vi "TextIcon.vi"(0 "Text":u32(colorbox)=6589059, 1 "picture":picture, 5 "Text":string, 7 "[user-specified font]":T1={"Font Name:"="Arial", "Size"=6, "Strikeout?"=FALSE, "Italic?"=FALSE, "Underline?"=FALSE, "Outline?"=FALSE, "Shadow?"=FALSE, "Bold?"=FALSE}, 9 "rect":T3={"left"=2, "top"=17, "right"=32, "bottom"=32}, 11 "error in (no error)":errorcluster, 12 "BG color(transparent)":u32(colorbox)=16777216) -> (4 ">> TextIcon >>":T4 caption="用户图层", 15 "error out":errorcluster)   [LabVIEW 2015]
uses:
  <vilib>/LabVIEW Icon API/API_User Layer Data.ctl
  <vilib>/Utility/miscctls.llb/LVPoint32TypeDef.ctl
  <vilib>/picture/picture.llb/imagedata.ctl
  1_ctl/Ctl-Text-Set.ctl
  1_ctl/ctl-font.ctl
  <vilib>/LabVIEW Icon API/LabVIEW Icon API.lvlib
panel:
  out "picture 2":picture
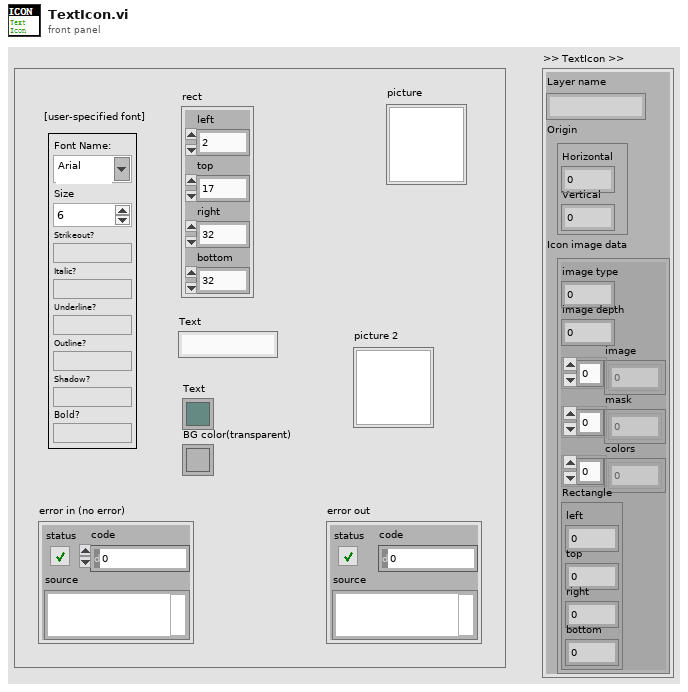
[diagram p1: front panel]
types:
  T1 = typedef "Ctl-Text-Set.ctl" = cluster{"Font Name:":T2, "Size":i16, "Strikeout?":bool, "Italic?":bool, "Underline?":bool, "Outline?":bool, "Shadow?":bool, "Bold?":bool}
  T2 = typedef "ctl-font.ctl" = string
  T3 = cluster{"left":i16, "top":i16, "right":i16, "bottom":i16}
  T4 = typedef "LabVIEW Icon API.lvlib/API_User Layer Data.ctl" = cluster{"Layer name":string, "Origin":T5, "Icon image data":T6}
  T5 = typedef "LVPoint32TypeDef.ctl" = cluster{"Horizontal":i32, "Vertical":i32}
  T6 = typedef "imagedata.ctl" = cluster{"image type":i32, "image depth":i32, "image":u8[], "mask":u8[], "colors":u32[], "Rectangle":cluster{"left":i16, "top":i16, "right":i16, "bottom":i16}}
  T7 = enum16{"User-specified Font", "Application Font", "System Font", "Dialog Font"}
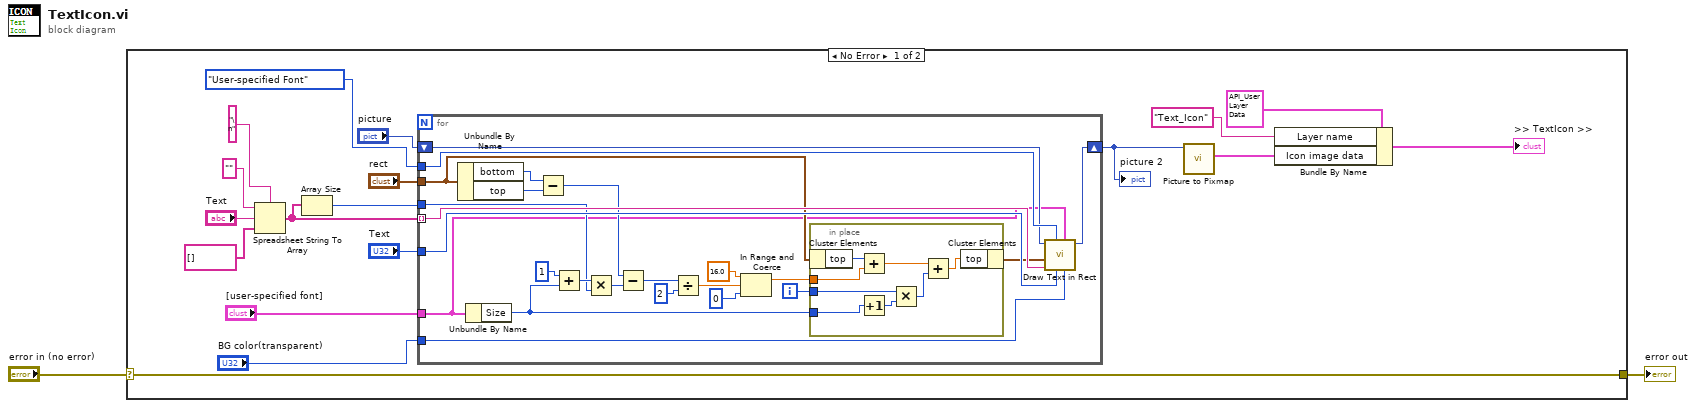
[diagram p0: block diagram]
diagram:
  n1 = case shown="No Error" "error in (no error)" {
    selector: "error in (no error)" -> [w7 w53]
    tunnel: [w7 w53] -> w1
    frame No Error {
      n2 = Spreadsheet String To Array(delimiter (Tab)="\n", format string="", spreadsheet string="Text", array type (2D Dbl)=string[] []) -> (array=w6:string[])
      n3 = Array Size(array=w6) -> (size(s)=w5:i32)
      n4 = for {
        tunnel: "Text" -> [w43]
        tunnel: "BG color(transparent)" -> [w42]
        tunnel: T7."User-specified Font" ("desired font(Application)") -> [w41]
        tunnel: "[user-specified font]" -> [w21]
        shift-right: [w44] -> w4
        shift-left: "picture" -> [w40]
        tunnel: w6 -> [w39] mode=indexing
        tunnel: "rect" -> [w36]
        tunnel: w5 -> [w29]
        i -> [w37]
        n5 = Unbundle By Name(w36) -> ("bottom"=w35:i16, "top"=w34:i16)
        n6 = Unbundle By Name(w21) -> ("Size"=w32:i16)
        n7 = Subtract(x=w35, y=w34) -> (x-y=w33:i16)
        n8 = Add(x=i16 1, y=w32) -> (x+y=w30:i16)
        n9 = Multiply(x=w30, y=w29) -> (x*y=w28:i32)
        n10 = Subtract(x=w33, y=w28) -> (x-y=w27:i32)
        n11 = Divide(x=w27, y=2) -> (x/y=w24:dbl)
        n12 = In Range and Coerce(upper limit=16.0, x=w24, lower limit=0 ("y")) -> (coerced(x)=w23:dbl)  [unwired: 1 out]
        n13 = in-place {
          in-place-border: w37 -> [w52]
          in-place-border: w32 -> [w50]
          in-place-border: w23 -> [w48]
          n14 = in-place-cluster #1(w36) -> ("top"=w46:i16)
          n15 = Add(x=w46, y=w48) -> (x+y=w47:dbl)
          n16 = Increment(x=w50) -> (x+1=w49:i16)
          n17 = Multiply(x=w52, y=w49) -> (x*y=w51:i32)
          n18 = Add(x=w47, y=w51) -> (x+y=w45:dbl)
          n19 = in-place-cluster #1("top"=w45) -> (w38:T3)
        }
        n20 = call <vilib>:"Draw Text in Rect.vi"("BG color(transparent)"=w42, "[user-specified font]"=w21, "text color(black)"=w43, "desired font(Application)"=w41, "text"=w39, "rect"=w38, "picture"=w40) -> ("new picture"=w44:picture)  [unwired: 4 in]
      }
      "picture 2" <- w4
      n21 = call <vilib>:"Picture to Pixmap.vi"("picture"=w4) -> ("image data"=w19:T6)  [unwired: 9 in, 1 out]
      n22 = Bundle By Name(cluster=T4 {"Layer name"="", "Origin"={"Horizontal"=0, "Vertical"=0}, "Icon image data"={"image type"=0, "image depth"=0, "image"=[], "mask"=[], "colors"=[], "Rectangle"={"left"=0, "top"=0, "right"=0, "bottom"=0}}} ("User layer"), "Layer name"="Text_Icon", "Icon image data"=w19) -> (→">> TextIcon >>":T4)
    }
    frame Error {
    }
  }
  "error out" <- w1
